vi "Kinetic energy from voltage.vi"(10 "Module Voltage":dbl) -> (2 "Kinetic Energy from voltage":dbl)   [LabVIEW 2020]
doc: "This SubVi is prototype."
panel:
  # "PROTOTYPE"
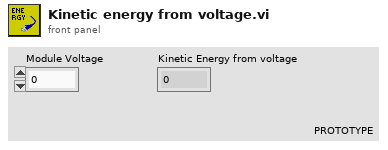
[diagram p1: front panel]
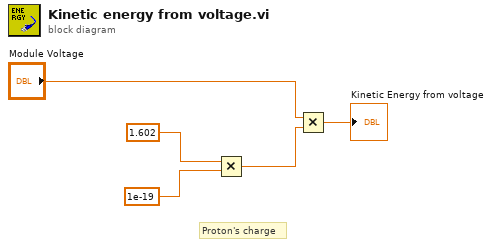
[diagram p0: block diagram]
diagram:
  # "Proton's charge"
  n1 = Multiply(x=1.602, y=1e-19) -> (x*y=w4:dbl)
  n2 = Multiply(x="Module Voltage", y=w4) -> (x*y=→"Kinetic Energy from voltage":dbl)
